vi "SetAttributeViInt32_CP_Monitor_PS_Waveform.vi"(7 "AttributeValue":i32 format="%.0g", 8 "error in (no error)":errorcluster {"code" format="%.0x"}, 9 "AttributeID":u32(ring)=1150050 items=["CHANNELPOWER_AVERAGE_COUNT"=1150050, "CHANNELPOWER_AVERAGE_MODE"=1190231, "CHANNELPOWER_DETECTOR_TYPE"=1150035, "CHANNELPOWER_DISPLAY_WINDOWY_REF_POSITION"=1190658, "CHANNELPOWER_FREQUENCY_PHASE_NOISE_OPTION_STATE"=1190660, "CHANNELPOWER_MARKER_ACTIVE_MARKER"=1190249, "CHANNELPOWER_MARKER_DELTA_REFERENCE"=1190252, "CHANNELPOWER_MARKER_TYPE"=1190255, "CHANNELPOWER_POWER_SPECTRAL_DENSITY_REFERENCE"=1150108, "CHANNELPOWER_SWEEPCOUPLING_BANDWIDTH_SHAPE"=1190251, "CHANNELPOWER_SWEEPCOUPLING_SWEEP_POINTS"=1190258, "CHANNELPOWER_SWEEPCOUPLING_SWEEP_TIME_AUTO_RULES"=1190261, "CHANNELPOWER_TRACE_TYPE"=1150106, "CHANNELPOWER_TRIGGER_SOURCE"=1150021, "MONITOR_AVERAGE_COUNT"=1190348, "MONITOR_AVERAGE_MODE"=1190350, "MONITOR_DISPLAY_REF_POSITION"=1191496, "MONITOR_MARKER_ACTIVE_MARKER"=1190368, "MONITOR_MARKER_DELTA_REFERENCE"=1190372, "MONITOR_MARKER_FUNCTION"=1190375, "MONITOR_MARKER_TRACE"=1150112, "MONITOR_MARKER_TYPE"=1190566, "MONITOR_SWEEPCOUPLING_SWEEP_POINTS"=1190362, "MONITOR_TRACE_DETECTOR_TYPE"=1190346, "MONITOR_TRACE_TYPE"=1190034, "MONITOR_TRIGGER_SOURCE"=1150022, "POWER_STATISTICS_MARKER_ACTIVE_MARKER"=1190423, "POWER_STATISTICS_MARKER_DELTA_REFERENCE"=1190427, "POWER_STATISTICS_MARKER_TRACE"=1190430, "POWER_STATISTICS_MARKER_TYPE"=1190582, "POWER_STATISTICS_SAMPLING_COUNT"=1190422, "POWER_STATISTICS_SWEEP_COUPLING_SWEEP_CYCLES"=1150110, "POWER_STATISTICS_TRIGGER_SOURCE"=1150056, "WAVEFORM_AVERAGE_COUNT"=1190537, "WAVEFORM_AVERAGE_MODE"=1190539, "WAVEFORM_AVERAGE_TIME_AVERAGE_COUNT"=1191502, "WAVEFORM_AVERAGE_TYPE"=1190540, "WAVEFORM_DISPLAY_IQWAVEFORM_VIEW_WINDOWX_REF_POSITION"=1191574, "WAVEFORM_DISPLAY_IQWAVEFORM_VIEW_WINDOWY_REF_POSITION"=1191578, "WAVEFORM_DISPLAY_VIEW"=1190544, "WAVEFORM_DISPLAY_VIEW_BY_NAME"=1150127, "WAVEFORM_DISPLAY_WINDOWX_REF_POSITION"=1191504, "WAVEFORM_DISPLAY_WINDOWY_REF_POSITION"=1191582, "WAVEFORM_FILTER_TYPE"=1191500, "WAVEFORM_FREQUENCY_SYNTHESIS_STATE"=1191508, "WAVEFORM_IF_GAIN"=1190531, "WAVEFORM_MARKER_ACTIVE_MARKER"=1190551, "WAVEFORM_MARKER_DELTA_REFERENCE"=1190555, "WAVEFORM_MARKER_FUNCTION"=1190557, "WAVEFORM_MARKER_TRACE"=1150126, "WAVEFORM_MARKER_TYPE"=1190586, "WAVEFORM_TRIGGER_SOURCE"=1150076], 10 "RepCapIdentifier":string, 11 "instrument handle":refnum<k15>) -> (0 "error out":errorcluster {"code" format="%.0x"}, 3 "instrument handle out":refnum<k15>)   [LabVIEW 2021, in "Keysight XSAnVMA.lvlib"]
doc: "Sets Int32 Attribute from instrumrnt driver.\nThe following attributes are supported:\n\nCHANNELPOWER_AVERAGE_COUNT\nCHANNELPOWER_AVERAGE_MODE\nCHANNELPOWER_DETECTOR_TYPE\nCHANNELPOWER_DISPLAY_WINDOWY_REF_POSITION\nCHANNELPOWER_FREQUENCY_PHASE_NOISE_OPTION_STATE\nCHANNELPOWER_MARKER_ACTIVE_MARKER\nCHANNELPOWER_MARKER_DELTA_REFERENCE\nCHANNELPOWER_MARKER_TYPE\nCHANNELPOWER_POWER_SPECTRAL_DENSITY_REFERENCE\nCHANNELPOWER_SWEEPCOUPLING_BANDWIDTH_SHAPE\nCHANNELPOWER_SWEEPCOUPLING_SWEEP_POINTS\nCHANNELPOWER_SWEEPCOUPLING_SWEEP_TIME_AUTO_RULES\nCHANNELPOWER_TRACE_TYPE\nCHANNELPOWER_TRIGGER_SOURCE\nMONITOR_AVERAGE_COUNT\nMONITOR_AVERAGE_MODE\nMONITOR_DISPLAY_REF_POSITION\nMONITOR_MARKER_ACTIVE_MARKER\nMONITOR_MARKER_DELTA_REFERENCE\nMONITOR_MARKER_FUNCTION\nMONITOR_MARKER_TRACE\nMONITOR_MARKER_TYPE\nMONITOR_SWEEPCOUPLING_SWEEP_POINTS\nMONITOR_TRACE_DETECTOR_TYPE\nMONITOR_TRACE_TYPE\nMONITOR_TRIGGER_SOURCE\nPOWER_STATISTICS_MARKER_ACTIVE_MARKER\nPOWER_STATISTICS_MARKER_DELTA_REFERENCE\nPOWER_STATISTICS_MARKER_TRACE\nPOWER_STATISTICS_MARKER_TYPE\nPOWER_STATISTICS_SAMPLING_COUNT\nPOWER_STATISTICS_SWEEP_COUPLING_SWEEP_CYCLES\nPOWER_STATISTICS_TRIGGER_SOURCE\nWAVEFORM_AVERAGE_COUNT\nWAVEFORM_AVERAGE_MODE\nWAVEFORM_AVERAGE_TIME_AVERAGE_COUNT\nWAVEFORM_AVERAGE_TYPE\nWAVEFORM_DISPLAY_IQWAVEFORM_VIEW_WINDOWX_REF_POSITION\nWAVEFORM_DISPLAY_IQWAVEFORM_VIEW_WINDOWY_REF_POSITION\nWAVEFORM_DISPLAY_VIEW\nWAVEFORM_DISPLAY_VIEW_BY_NAME\nWAVEFORM_DISPLAY_WINDOWX_REF_POSITION\nWAVEFORM_DISPLAY_WINDOWY_REF_POSITION\nWAVEFORM_FILTER_TYPE\nWAVEFORM_FREQUENCY_SYNTHESIS_STATE\nWAVEFORM_IF_GAIN\nWAVEFORM_MARKER_ACTIVE_MARKER\nWAVEFORM_MARKER_DELTA_REFERENCE\nWAVEFORM_MARKER_FUNCTION\nWAVEFORM_MARKER_TRACE\nWAVEFORM_MARKER_TYPE\nWAVEFORM_TRIGGER_SOURCE"
uses:
  <instrlib>/Keysight XSAnVMA/Keysight XSAnVMA.lvlib
  KtXSAnVMA_64.dll
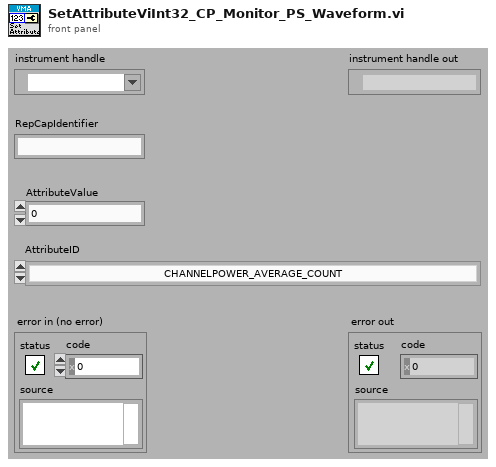
[diagram p1: front panel]
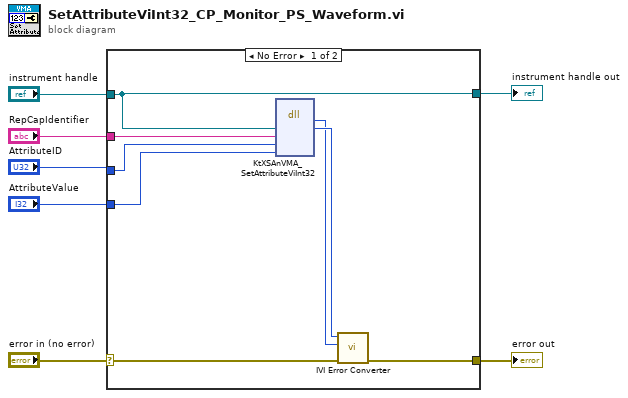
[diagram p0: block diagram]
diagram:
  n1 = case shown="No Error" "error in (no error)" {
    selector: "error in (no error)" -> [w13 w17]
    tunnel: [w12 w17] -> w7
    tunnel: "instrument handle" -> [w8 w16]
    tunnel: "RepCapIdentifier" -> [w11 _]
    tunnel: "AttributeID" -> [w10 _]
    tunnel: "AttributeValue" -> [w9 _]
    tunnel: [w8 w16] -> w1
    frame No Error {
      n2 = dll-call lib="KtXSAnVMA**.dll" fn="KtXSAnVMA_SetAttributeViInt32"("Vi"=w8, "RepCapIdentifier"=w11, "AttributeID"=w10, "AttributeValue"=w9) -> ("return type"=w14:i32, "Vi"=w15:u32)  [unwired: 6 in, 2 out]
      n3 = call <instrlib>:"IVI Error Converter.vi"("error in (no error)"=w13, "IVI error code (0)"=w14, "instrument handle"=w15) -> ("error out"=w12:errorcluster)  [unwired: 7 in, 1 out]
    }
    frame Error {
    }
  }
  "error out" <- w7
  "instrument handle out" <- w1
